vi "Fit Control to Tab.vi"(5 "Control":refnum<vi>, 6 "error in (no error)":errorcluster, 8 "Margin":T2={"Left"=8, "Right"=8, "Top"=8, "Bottom"=8}, 9 "TabRef":refnum<vi>) -> (0 "error out":errorcluster, 1 "Rect":T1={"Left"=8, "Right"=8, "Height"=8, "Width"=8}, 3 "TabRef (dup)":refnum<vi>)   [LabVIEW 2017, in "csm-ui-support.lvlib"]
uses:
  csm-ui-support.lvlib
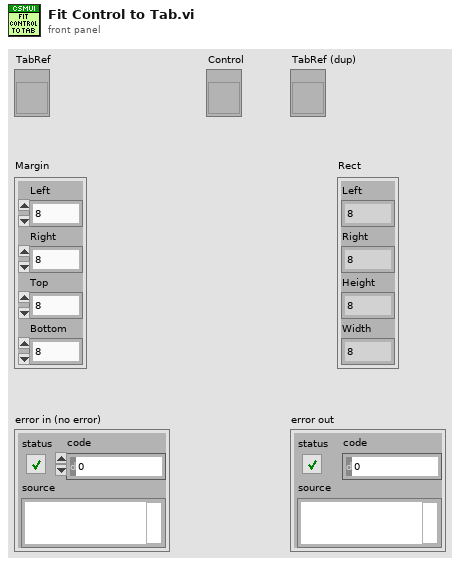
[diagram p1: front panel]
types:
  T1 = cluster{"Left":i32, "Right":i32, "Height":i32, "Width":i32}
  T2 = cluster{"Left":i32, "Right":i32, "Top":i32, "Bottom":i32}
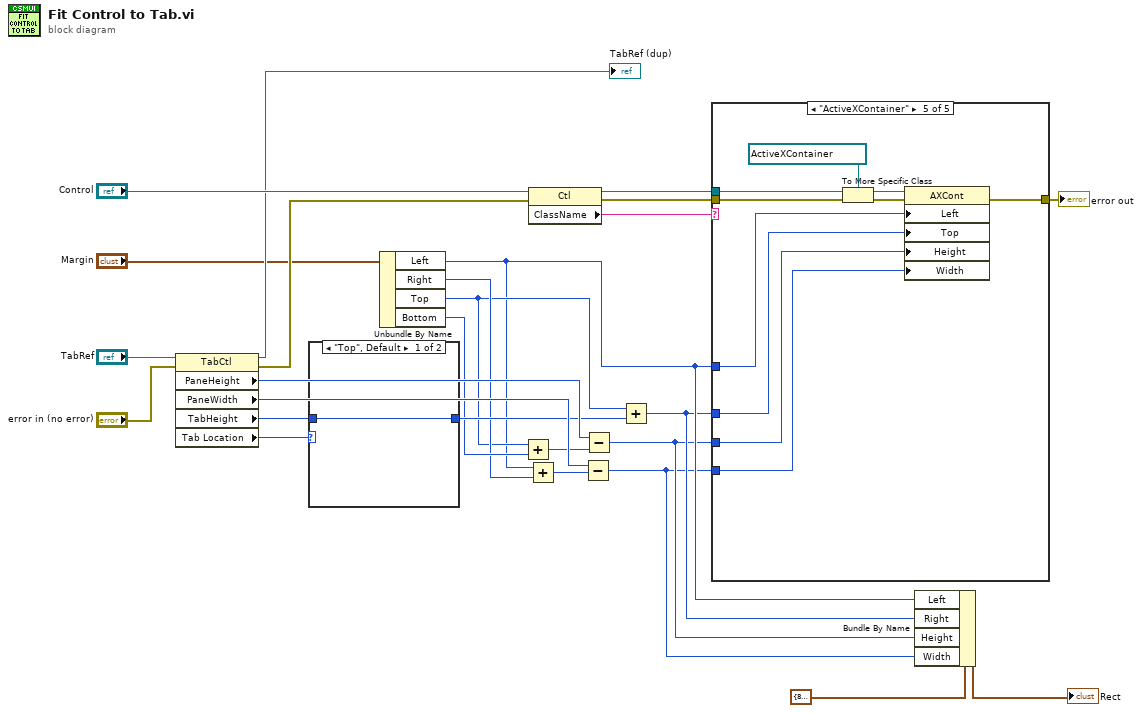
[diagram p0: block diagram]
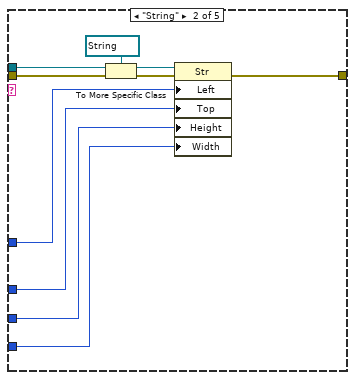
[diagram p3: hidden frame]
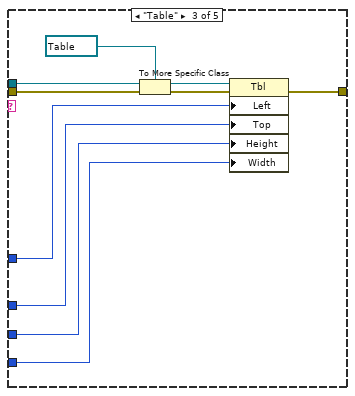
[diagram p4: hidden frame]
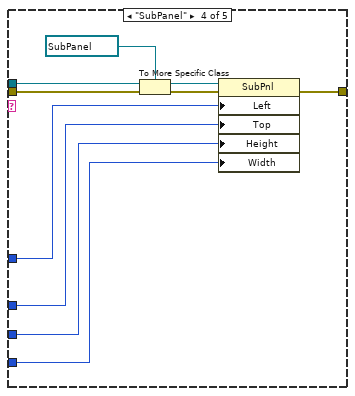
[diagram p5: hidden frame]
diagram:
  n1 = property class="TabCtl"(reference="TabRef", error in="error in (no error)") -> (reference out=→"TabRef (dup)":refnum<vi>, error out=w17:errorcluster, "PaneHeight"=w26:u32, "PaneWidth"=w25:u32, "TabHeight"=w22:u32, "Tab Location"=w24:enum32{"Top", "Bottom", "Left", "Right"})
  n2 = case shown="\"Top\", Default" w24 {
    tunnel: [w27 _] -> w23
    tunnel: w22 -> [w27 _]
    frame "Top", Default {
    }
    frame "Bottom" {
    }
  }
  n3 = Unbundle By Name("Margin") -> ("Left"=w4:i32, "Right"=w9:i32, "Top"=w7:i32, "Bottom"=w11:i32)
  n4 = Add(x=w7, y=w11) -> (x+y=w10:i32)
  n5 = Add(x=w4, y=w9) -> (x+y=w8:i32)
  n6 = property class="Ctl"(reference="Control", error in=w17) -> (reference out=w21:refnum<vi>, error out=w20:errorcluster, "ClassName"=w19:string)
  n7 = Subtract(x=w25, y=w8) -> (x-y=w1:u32)
  n8 = Subtract(x=w26, y=w10) -> (x-y=w2:u32)
  n9 = Add(x=w7, y=w23) -> (x+y=w3:u32)
  n10 = case shown="\"ActiveXContainer\"" w19 {
    tunnel: w4 -> [_ w38 w46 w56 w66]
    tunnel: w3 -> [_ w37 w45 w55 w65]
    tunnel: w2 -> [_ w36 w44 w54 w64]
    tunnel: w1 -> [_ w35 w43 w53 w63]
    tunnel: w21 -> [_ w34 w48 w58 w68]
    tunnel: w20 -> [w28 w33 w47 w57 w67]
    tunnel: [w28 w29 w40 w50 w60] -> w15
    frame Default {
    }
    frame "String" {
      n11 = To More Specific Class(target class=refnum<vi> refnum ("Error History"), reference=w34, error in=w33) -> (specific class reference=w32:refnum<vi>, error out=w30:errorcluster)
      n12 = property class="Str"(reference=w32, error in=w30, "Left"=w38, "Top"=w37, "Height"=w36, "Width"=w35) -> (error out=w29:errorcluster)  [unwired: 1 out]
    }
    frame "Table" {
      n13 = To More Specific Class(target class=refnum<vi> refnum ("Broadcast Registry"), reference=w48, error in=w47) -> (specific class reference=w41:refnum<vi>, error out=w42:errorcluster)
      n14 = property class="Tbl"(reference=w41, error in=w42, "Left"=w46, "Top"=w45, "Height"=w44, "Width"=w43) -> (error out=w40:errorcluster)  [unwired: 1 out]
    }
    frame "SubPanel" {
      n15 = To More Specific Class(target class=refnum<vi> refnum ("Broadcast Registry"), reference=w58, error in=w57) -> (specific class reference=w51:refnum<vi>, error out=w52:errorcluster)
      n16 = property class="SubPnl"(reference=w51, error in=w52, "Left"=w56, "Top"=w55, "Height"=w54, "Width"=w53) -> (error out=w50:errorcluster)  [unwired: 1 out]
    }
    frame "ActiveXContainer" {
      n17 = To More Specific Class(target class=refnum<vi> refnum ("Broadcast Registry"), reference=w68, error in=w67) -> (specific class reference=w61:refnum<vi>, error out=w62:errorcluster)
      n18 = property class="AXCont"(reference=w61, error in=w62, "Left"=w66, "Top"=w65, "Height"=w64, "Width"=w63) -> (error out=w60:errorcluster)  [unwired: 1 out]
    }
  }
  "error out" <- w15
  n19 = Bundle By Name(cluster=T1 {"Left"=8, "Right"=8, "Height"=8, "Width"=8} ("Rect"), "Left"=w4, "Right"=w3, "Height"=w2, "Width"=w1) -> (→"Rect":T1)
